vi "checkForceST.vi"(8 "error in (no error)":errorcluster, 11 "Model in":refnum<class "Model.lvclass">) -> (0 "error out":errorcluster, 2 "reachedForceTriggerIsTrue":bool, 3 "Model out":refnum<class "Model.lvclass">)   [LabVIEW 2015, in "Model.lvclass"]
uses:
  Model.lvclass
  Model.lvclass/Model.ctl
  <userlib>/Common/Devices/ForceSensorCalculator/ForceSensorCalculator/ForceSensorCalculator.lvclass/ForceSensorCalculator.ctl
  ApplicationElements/SystemController/SystemController.lvclass
  <userlib>/Common/Devices/ForceSensorCalculator/ForceSensorCalculator/ForceSensorCalculator.lvclass
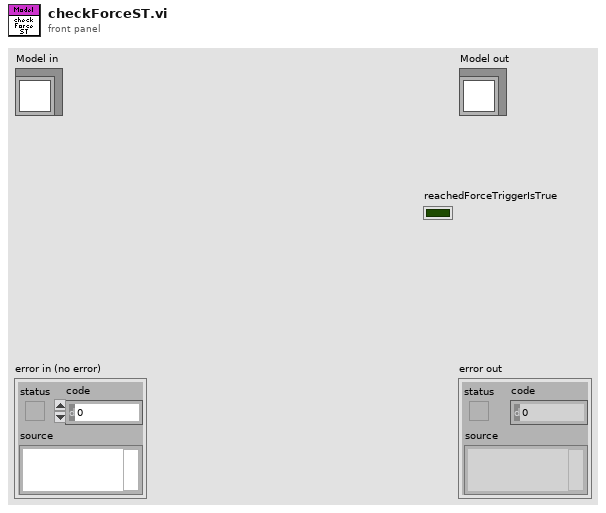
[diagram p1: front panel]
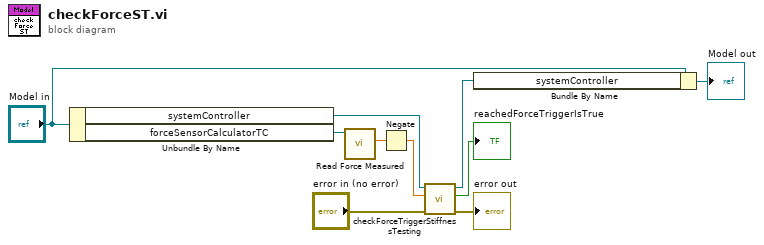
[diagram p0: block diagram]
diagram:
  n1 = Unbundle By Name("Model in") -> ("systemController"=w8:refnum<class "SystemController.lvclass">, "forceSensorCalculatorTC"=w3:refnum<class "ForceSensorCalculatorTC.lvclass">)
  n2 = call <userlib>:"Read Force Measured.vi"("ForceSensor in"=w3) -> ("Force Demand"=w2:dbl[unit])  [unwired: 9 in, 1 out]
  n3 = Negate(x=w2) -> (-x=w1:dbl[unit])
  n4 = call "checkForceTriggerStiffnessTesting.vi"("error in (no error)"="error in (no error)", "Force Measured"=w1, "SystemController in"=w8) -> ("error out"=→"error out":errorcluster, "forceTriggerReached"=→"reachedForceTriggerIsTrue":bool, "SystemController out"=w7:refnum<class "SystemController.lvclass">)  [unwired: 6 in]
  n5 = Bundle By Name(cluster="Model in", "systemController"=w7) -> (→"Model out":refnum<class "Model.lvclass">)
